vi "Lakeshore_get_temp.vi"(0 "VISA resource name":refnum<visa-resource-name>, 1 "Lakeshore Delay":u32, 5 "Desired Sensor":T1, 11 "error in (no error)":errorcluster) -> (4 "VISA resource name out":refnum<visa-resource-name>, 6 "Lakeshore_Resist":dbl, 10 "Lakeshore Level Read Status":bool, 15 "error out":errorcluster)   [LabVIEW 2018]
uses:
  <vilib>/Utility/error.llb/whitespace.ctl
  sensor_select.ctl
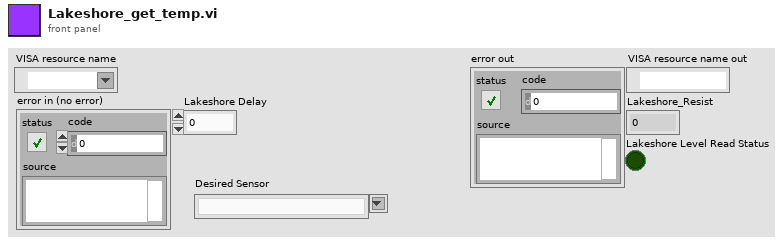
[diagram p1: front panel]
types:
  T1 = typedef "sensor_select.ctl" = string
  T2 = typedef "whitespace.ctl" = u16
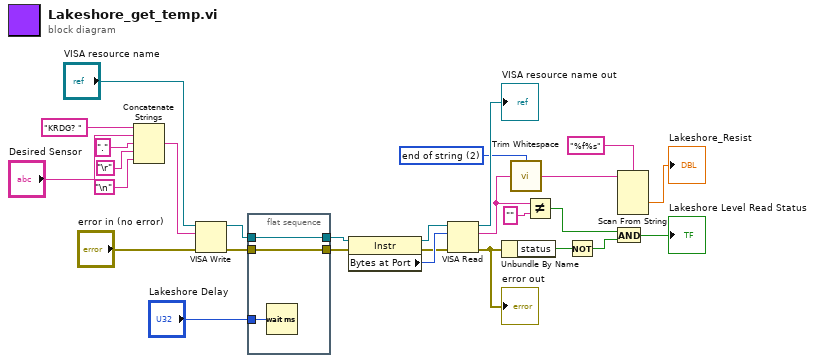
[diagram p0: block diagram]
diagram:
  w15 = T2 2 items=["both", "start of string", "end of string"] ("location (both)")
  n1 = Concatenate Strings("KRDG? " ("string"), "Desired Sensor", "." ("string"), "\r", "\n") -> (w25:string)
  n2 = VISA Write(VISA resource name="VISA resource name", write buffer=w25, error in (no error)="error in (no error)") -> (VISA resource name out=w24:refnum<visa-resource-name>, error out=w23:errorcluster)  [unwired: 1 out]
  n3 = flat-sequence {
    tunnel: w24 -> [w30]
    tunnel: w23 -> [w31]
    tunnel: [w31] -> w20
    tunnel: [w30] -> w21
    tunnel: "Lakeshore Delay" -> [w29]
    frame #0 {
      n4 = Wait (ms)(milliseconds to wait=w29) -> ()  [unwired: 1 out]
    }
  }
  n5 = property class="Instr"(reference=w21, error in=w20) -> (reference out=w19:refnum<visa-resource-name>, error out=w17:errorcluster, "Bytes at Port"=w18:u32)
  n6 = VISA Read(VISA resource name=w19, byte count=w18, error in (no error)=w17) -> (VISA resource name out=→"VISA resource name out":refnum<visa-resource-name>, read buffer=w4:string, error out=w11:errorcluster)  [unwired: 1 out]
  "error out" <- w11
  n7 = Unbundle By Name(w11) -> ("status"=w10:bool)
  n8 = call <vilib>:"Trim Whitespace.vi"("string"=w4, "location (both)"=w15) -> ("trimmed string"=w14:string)
  n9 = Not Equal?(x=w4, y="") -> (x != y?=w7:bool)
  n10 = Not(x=w10) -> (.not. x?=w8:bool)
  n11 = And(x=w7, y=w8) -> (x .and. y?=→"Lakeshore Level Read Status":bool)
  n12 = Scan From String(format string="%f%s", input string=w14) -> (output 1=→"Lakeshore_Resist":dbl)  [unwired: 5 in, 3 out]
